vi "Status Array V.I.G.vi"(7 "VI Action":T1, 10 "index":i32, 11 "Element":bool) -> (3 "Array":bool[](array[boolean]))   [LabVIEW 2010]
uses:
  status action.ctl
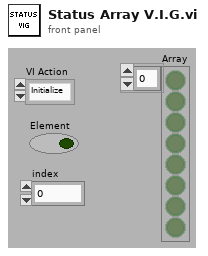
[diagram p1: front panel]
types:
  T1 = typedef "status action.ctl" = enum16{"Initialize", "Write", "Read"}
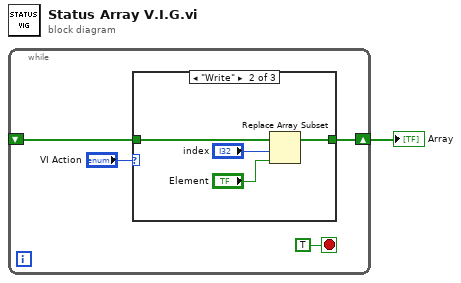
[diagram p0: block diagram]
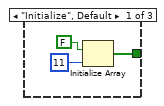
[diagram p2: hidden frame]
diagram:
  n1 = while {
    shift-right: [w3] -> w1
    shift-left: _ -> [w4]
    stop <- TRUE stop-if-true
    n2 = case shown="\"Write\"" "VI Action" {
      tunnel: w4 -> [_ w12 w13]
      tunnel: [w7 w11 w13] -> w3
      frame "Initialize", Default {
        n3 = Initialize Array(FALSE, 11 ("dimension size")) -> (w7:bool[])
      }
      frame "Write" {
        n4 = Replace Array Subset(array=w12, new element="Element", index="index") -> (w11:bool[])
      }
      frame "Read" {
      }
    }
  }
  "Array" <- w1
